vi "match bounding box area.vi"(1 "particle measurements (bounding box)":dbl[][](array[numeric]), 2 "bounding box in":dbl[](array[numeric])) -> (0 "matching bounding box":dbl[](array[numeric]))   [LabVIEW 2014]
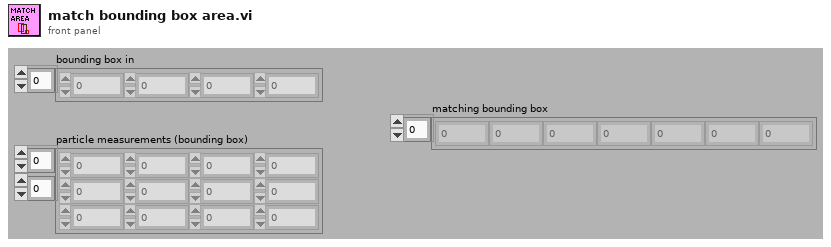
[diagram p1: front panel]
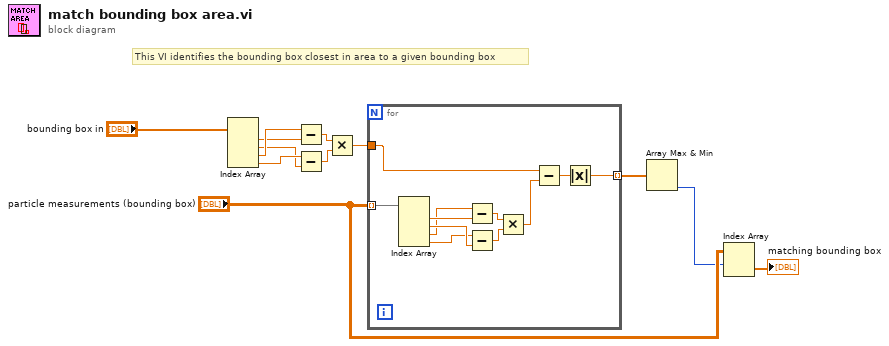
[diagram p0: block diagram]
diagram:
  # "This VI identifies the bounding box closest in area to a given bounding box"
  n1 = Index Array(array="bounding box in") -> (element #1=w11:dbl, element #2=w9:dbl, element #3=w12:dbl, element #4=w10:dbl)  [unwired: 4 in]
  n2 = Subtract(x=w12, y=w11) -> (x-y=w8:dbl)
  n3 = Subtract(x=w10, y=w9) -> (x-y=w7:dbl)
  n4 = Multiply(x=w8, y=w7) -> (x*y=w5:dbl)
  n5 = for {
    tunnel: "particle measurements (bounding box)" -> [w17] mode=indexing
    tunnel: w5 -> [w16]
    tunnel: [w13] -> w4 mode=indexing
    n6 = Index Array(array=w17) -> (element #1=w19:dbl, element #2=w21:dbl, element #3=w18:dbl, element #4=w20:dbl)  [unwired: 4 in]
    n7 = Subtract(x=w18, y=w19) -> (x-y=w22:dbl)
    n8 = Subtract(x=w20, y=w21) -> (x-y=w23:dbl)
    n9 = Multiply(x=w22, y=w23) -> (x*y=w15:dbl)
    n10 = Subtract(x=w16, y=w15) -> (x-y=w14:dbl)
    n11 = Absolute Value(x=w14) -> (abs(x)=w13:dbl)
  }
  n12 = Array Max & Min(array=w4) -> (min index (indices)=w2:i32)  [unwired: 3 out]
  n13 = Index Array(array="particle measurements (bounding box)", index (row)=w2) -> (element=→"matching bounding box":dbl[])  [unwired: 1 in]
